vi "get_device_list.vi"(11 "error in (no error)":errorcluster) -> (6 "device_list":string[][](array[string]), 15 "error out":errorcluster)   [LabVIEW 2012]
doc: "Retrieves a 2-D list (array) of connected devices.\n\ncolumn[0] = Device Index\ncolumn[1] = Serial Number\ncolumn[2] = Description\n\nProduced By:\n\nChristopher Lemieux\nKod Integrations, LLC\n4835 Marianne Drive\nMount Airy, MD 21771\nhttp://www.kodintegrations.com\nemail: clemieux@kodintegrations.com\nphone: (240) 687-1288"
uses:
  controls/info_options.ctl
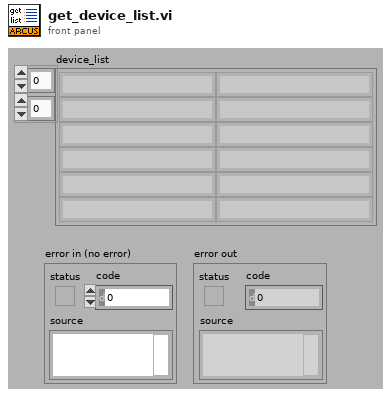
[diagram p1: front panel]
types:
  T1 = typedef "info_options.ctl" = enum16{"device_name", "description"}
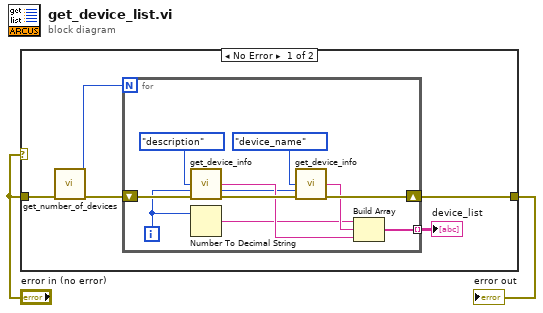
[diagram p0: block diagram]
diagram:
  n1 = case shown="No Error" "error in (no error)" {
    tunnel: "error in (no error)" -> [w5 w18]
    tunnel: [w4 w18] -> w1
    frame No Error {
      n2 = call "get_number_of_devices.vi"("error in (no error)"=w5) -> ("num_of_devices (out)"=w7:i32, "error out"=w6:errorcluster)  [unwired: 13 in]
      n3 = for {
        N: w7 -> [_]
        shift-right: [w13] -> w4
        shift-left: w6 -> [w17]
        tunnel: [w10] -> w3 mode=indexing
        i -> [w9]
        n4 = call "get_device_info.vi"("info_options"=info_options."description", "device_index"=w9, "error in (no error)"=w17) -> ("retrieved_info (str)"=w11:string, "error out"=w14:errorcluster)  [unwired: 11 in]
        n5 = Number To Decimal String(number=w9) -> (decimal integer string=w8:string)  [unwired: 1 in]
        n6 = call "get_device_info.vi"("info_options"=info_options."device_name", "device_index"=w9, "error in (no error)"=w14) -> ("retrieved_info (str)"=w12:string, "error out"=w13:errorcluster)  [unwired: 11 in]
        n7 = Build Array(w8, w12, w11) -> (w10:string[])
      }
      "device_list" <- w3
    }
    frame Error {
    }
  }
  "error out" <- w1
